vi "Shift Threshold Calculation.vi"(1 "Throttle (%)":sgl, 2 "Gear":sgl) -> (9 "Up Threshold (mph)":sgl, 10 "Down Threshold (mph)":sgl)   [LabVIEW 2016, in "NI-PCG Vehicle Model.lvlib"]
uses:
  NI-PCG Vehicle Model.lvlib
  Globals/Parameters.vi
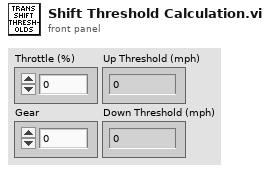
[diagram p1: front panel]
types:
  T1 = cluster{"XArray":sgl[], "YArray":sgl[], "ZArray":sgl[][]}
  T2 = typedef "NI-PCG Vehicle Model.lvlib/Engine Parameters.ctl" = cluster{"Ambient Parameters":cluster{"Temperature (K)":sgl, "Pressure (Pa)":sgl}, "Air Parameters":cluster{"R (Ideal Gas Constant)":sgl, "Molecular Weight":sgl, "Cp (Specific Heat Constant)":sgl, "Density (kg/m^3)":sgl, "Stoichiometric A/F Ratio":sgl}, "Engine Geometry Parameters":cluster{"Cylinder Volume (l)":sgl, "J (Rotational Moment of Inertia)":sgl, "Minimuim Engine Speed":sgl, "Maximum Engine Speed":sgl, "Intake Manifold Volume (l)":sgl}, "Volumetric Efficiency Map":cluster{"MAP":sgl[], "RPM":sgl[], "Table":sgl[][]}, "Fuel LHV (J/kg)":sgl, "Combustion Efficiency Map":cluster{"Spark Timing (deg BTDC))":sgl[], "Engine Speed (RPM)":sgl[], "Combustion Efficiency":sgl[][]}, "Thermodynamic Efficiency":sgl}
  T3 = typedef "NI-PCG Vehicle Model.lvlib/Transmission Parameters.ctl" = cluster{"Final Drive Ratio":sgl, "Transmission Gear Ratios":cluster{"Gears":sgl[], "Gear Ratios":sgl[]}, "Torque Converter Map":cluster{"Speed Ratio":sgl[], "K Factor":sgl[], "Torque Ratio":sgl[]}, "Upshift Throttle":sgl[], "Downshift Throttle":sgl[], "Upshift Table":sgl[][], "Downshift Table":sgl[][], "Wait Time":u8}
  T4 = typedef "NI-PCG Vehicle Model.lvlib/Vehicle Parameters.ctl" = cluster{"Vehicle Mass (kg)":sgl, "Vehicle Cd":sgl, "Vehicle Frontal Area (m^2)":sgl, "Wheel Radius (m)":sgl, "Wheel Rolling Resistance":sgl}
  T5 = cluster{"Engine Parameters":T2, "Transmission Parameters":T3, "Vehicle Parameters":T4}
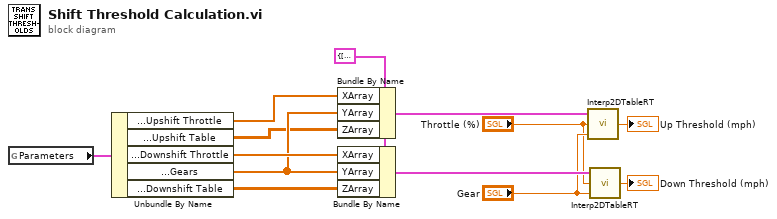
[diagram p0: block diagram]
diagram:
  w1 = T1 {"XArray"=[], "YArray"=[], "ZArray"=[]} ("2DTable")
  n1 = global read "Parameters.vi" "Parameters"() -> (w3:T5)
  n2 = Unbundle By Name(w3) -> ("Transmission Parameters.Upshift Throttle"=w13:sgl[], "Transmission Parameters.Upshift Table"=w8:sgl[][], "Transmission Parameters.Downshift Throttle"=w12:sgl[], "Transmission Parameters.Transmission Gear Ratios.Gears"=w11:sgl[], "Transmission Parameters.Downshift Table"=w10:sgl[][])
  n3 = Bundle By Name(cluster=w1, "XArray"=w13, "YArray"=w11, "ZArray"=w8) -> (w2:T1)
  n4 = Bundle By Name(cluster=w1, "XArray"=w12, "YArray"=w11, "ZArray"=w10) -> (w9:T1)
  n5 = call <vilib>:"Interp2DTableRT.vi"("Y"="Gear", "X"="Throttle (%)", "2DTable"=w2) -> ("Z"=→"Up Threshold (mph)":sgl)
  n6 = call <vilib>:"Interp2DTableRT.vi"("Y"="Gear", "X"="Throttle (%)", "2DTable"=w9) -> ("Z"=→"Down Threshold (mph)":sgl)
